vi "Keithley6485 Close.vi"(2 "error in":errorcluster, 3 "VISA in":refnum<visa-resource-name>="COM3") -> (0 "error out":errorcluster)   [LabVIEW 2018]
panel:
  in  "Exit configuration":string=":SYST:LOC"
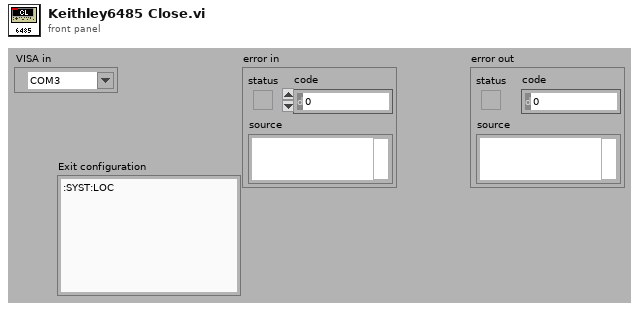
[diagram p1: front panel]
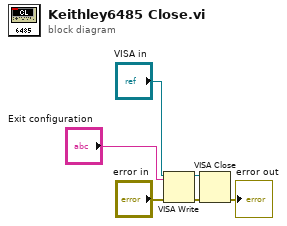
[diagram p0: block diagram]
diagram:
  n1 = VISA Write(VISA resource name="VISA in", write buffer="Exit configuration", error in (no error)="error in") -> (VISA resource name out=w4:refnum<visa-resource-name>, error out=w3:errorcluster)  [unwired: 1 out]
  n2 = VISA Close(VISA resource name=w4, error in (no error)=w3) -> (error out=→"error out":errorcluster)
